vi "Wait until done.vi"(8 "error in (no error)":errorcluster, 10 "Result Registration Refnum":T1, 11 "Execution API In":refnum<class "Execution API.lvclass">) -> (0 "error out":errorcluster, 2 "Output":string, 3 "Execution API Out":refnum<class "Execution API.lvclass">)   [LabVIEW 2020, in "Execution API.lvclass"]
doc: "Waits until all tests have been executed. The Result Events is obrained from the Register for Events.vi"
uses:
  Execution API.lvclass
  Result Types/Method Result/Method Result.ctl
  Result Types/Assertion Result/Public/TypeDefs/Status.ctl
  Result Types/Assertion Result/Assertion Result.ctl
  Result Types/Assertion Result/Public/TypeDefs/Assertion Type.ctl
  Result Types/Case Result/Test Case Result.ctl
  Result Types/Suite Results/Test Suite Result.ctl
  Result Types/Case Result/Private/Merge Status.vi
  Result Types/Case Result/Test Case Result.lvlib
  Result Types/Assertion Result/Assertion Result.lvlib
  Result Types/Method Result/Method Result.lvlib
  Result Types/Suite Results/Test Suite Result.lvlib
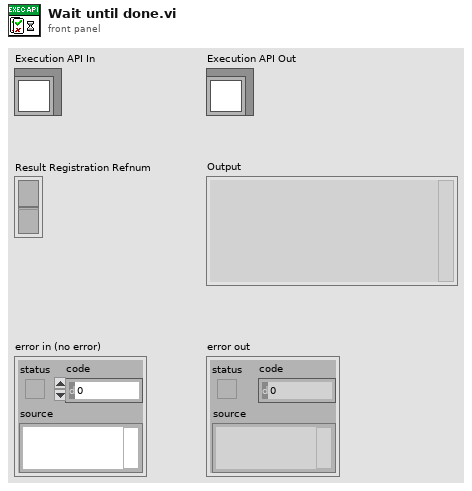
[diagram p1: front panel]
types:
  T1 = cluster{"Result Events":refnum<event-registration>, "Event Registration Refnum":refnum<event-registration>}
  T2 = typedef "Assertion Result.lvlib/Status.ctl" = enum16{"Pass", "Fail", "Error", "Skipped", "Setup Error", "Broken", "Teardown Error"}
  T3 = typedef "Test Case Result.lvlib/Test Case Result.ctl" = map{string, T4}
  T4 = typedef "Method Result.lvlib/Method Result.ctl" = cluster{"Test Case":string, "Test Method Name":string, "Status":T2, "Assertion Results":T5[], "Execution time":dbl, "Result String":string}
  T5 = typedef "Assertion Result.lvlib/Assertion Result.ctl" = cluster{"Status":T2, "Message":string, "Description":string, "Assertion Type":T6}
  T6 = typedef "Assertion Result.lvlib/Assertion Type.ctl" = enum16{"None", "Pass", "Fail", "Skip", "Pass if Equal", "Fail if Equal", "Pass if Error", "Fail if Error", "Pass if", "Fail if"}
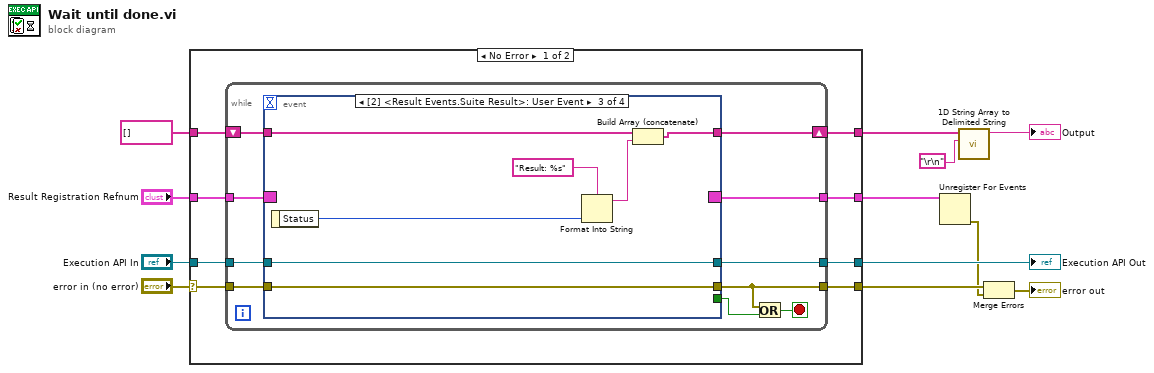
[diagram p0: block diagram]
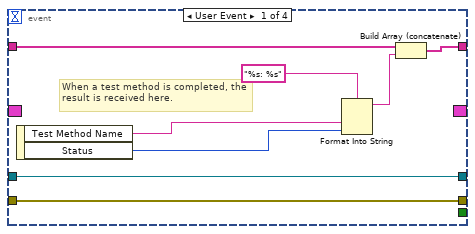
[diagram p2: hidden frame]
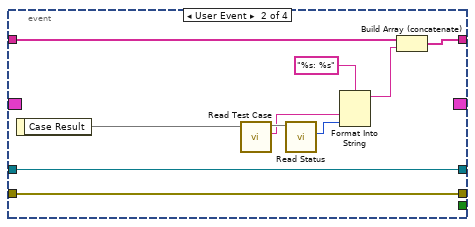
[diagram p3: hidden frame]
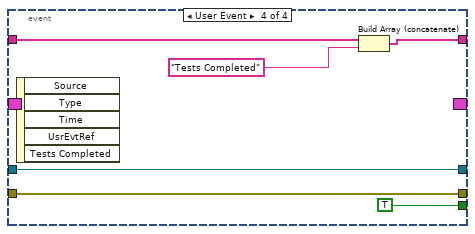
[diagram p4: hidden frame]
diagram:
  n1 = case shown="No Error" "error in (no error)" {
    selector: "error in (no error)" -> [w16 w65]
    tunnel: string[] [] -> [w20 w62]
    tunnel: [w19 w62] -> w11
    tunnel: "Execution API In" -> [w18 w64]
    tunnel: [w17 w64] -> w8
    tunnel: [w15 w65] -> w6
    tunnel: [w14 w63] -> w4
    tunnel: "Result Registration Refnum" -> [w13 w63]
    frame No Error {
      n2 = while {
        tunnel: w13 -> [w30]
        tunnel: w16 -> [w29]
        tunnel: w18 -> [w28]
        tunnel: [w26] -> w17
        tunnel: [w23] -> w15
        shift-right: [w22] -> w19
        shift-left: w20 -> [w25]
        tunnel: [w21] -> w14
        stop <- w24 stop-if-true
        n3 = event shown="[2] <Result Events.Suite Result>: User Event" {
          selector: w30 -> [_ _ _ _]
          dyn-events: [_ _ _ _] -> w21
          timeout: _ -> [_ _ _ _]
          tunnel: w29 -> [w32 w40 w50 w60]
          tunnel: w28 -> [w38 w48 w55 w61]
          tunnel: [_ _ _ TRUE] -> w27
          tunnel: [w38 w48 w55 w61] -> w26
          tunnel: [w32 w40 w50 w60] -> w23
          tunnel: w25 -> [w36 w46 w53 w58]
          tunnel: [w35 w45 w52 w57] -> w22
          event User Event {
            # "When a test method is completed, the result is received here."
            n4 = event-data() -> ("Test Method Name"=w33:string, "Status"=w31:T2)  [unwired: 1 in]
            n5 = Format Into String(format string="%s: %s", w33, w31) -> (resulting string=w34:string)  [unwired: 2 in, 1 out]
            n6 = Build Array (concatenate)(w36, w34) -> (w35:string[])
          }
          event User Event {
            n7 = event-data() -> ("Case Result"=w39:T3)  [unwired: 1 in]
            n8 = call "Read Test Case.vi"("Test Case Result In"=w39) -> ("Test Case"=w41:string, "Test Case Result Out"=w43:T3)  [unwired: 9 in]
            n9 = call "Read Status.vi"("Test Case Result In"=w43) -> ("Status"=w42:T2)  [unwired: 8 in, 2 out]
            n10 = Format Into String(format string="%s: %s", w41, w42) -> (resulting string=w44:string)  [unwired: 2 in, 1 out]
            n11 = Build Array (concatenate)(w46, w44) -> (w45:string[])
          }
          event User Event {
            n12 = event-data() -> ("Status"=w49:T2)  [unwired: 1 in]
            n13 = Format Into String(format string="Result: %s", w49) -> (resulting string=w51:string)  [unwired: 2 in, 1 out]
            n14 = Build Array (concatenate)(w53, w51) -> (w52:string[])
          }
          event User Event {
            n15 = event-data() -> ()  [unwired: 1 in, 5 out]
            n16 = Build Array (concatenate)(w58, "Tests Completed") -> (w57:string[])
          }
        }
        n17 = Or(x=w23, y=w27) -> (x .or. y?=w24:bool)
      }
    }
    frame Error {
    }
  }
  "Execution API Out" <- w8
  n18 = Unregister For Events(event registration refnum=w4) -> (error out=w2:errorcluster)  [unwired: 1 in]
  n19 = call <vilib>:"1D String Array to Delimited String.vi"("delimiter"="\r\n", "string array"=w11) -> ("delimited string"=→"Output":string)  [unwired: 9 in]
  n20 = Merge Errors(w6, w2) -> (→"error out":errorcluster)
